vi "AO init.vi"(8 "error in":errorcluster, 9 "Exposure duration specified (s)":dbl=0.5, 10 "Commands in":sgl[](array[numeric]), 11 "Matrix path":path=path "C:/Documents and Settings/User/Desktop/zw/20160113 200nm bead command matrix.aomc") -> (0 "error out":errorcluster, 1 "Camera":T2, 2 "Mirror":T5, 3 "Casao Matrix":T4, 4 "Haso":T3, 5 "Casao":T1)   [LabVIEW 2018]
uses:
  Casao LabVIEW SDK 1.0.5/Drivers_DPhaseModul/PhaseModul.ctl
  Casao LabVIEW SDK 1.0.5/Casao/CasaoMatrix/CasaoMatrix.ctl
  Casao LabVIEW SDK 1.0.5/Haso/Haso/Haso.ctl
  Casao LabVIEW SDK 1.0.5/Haso/Camera/Camera.ctl
  Casao LabVIEW SDK 1.0.5/Casao/Casao/Casao.ctl
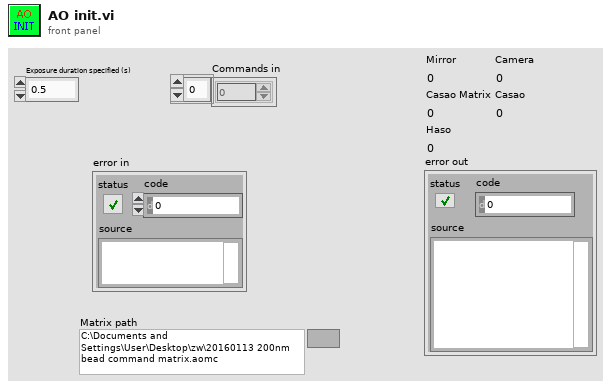
[diagram p1: front panel]
types:
  T1 = typedef "Casao.ctl" = i32
  T2 = typedef "Camera.ctl" = i32
  T3 = typedef "Haso.ctl" = i32
  T4 = typedef "CasaoMatrix.ctl" = i32
  T5 = typedef "PhaseModul.ctl" = i32
  T6 = typedef "Camera preferences.ctl" = cluster{"Exposure duration (µs)":u32, "Exposure duration specified (µs)":u32, "Number of summed images":u32, "Trigger type":enum16{"Internal", "TTL", "Software"}, "Trigger event":enum16{"falling", "rising"}, "Remove background image":bool, "Background image":T7, "Path to background image":string, "Auto exposure":bool, "Auto exposure target (%)":sgl, "Auto exposure tolerance (%)":sgl, "Timeout delay (ms)":u32, "Delay after trigger (µs)":i32}
  T7 = typedef "Image Compat.ctl" = cluster{"Signed/unsigned":bool, "Number of bits":T8, "Internal object id":i32, "Internal data id":i32}
  T8 = typedef "Data alignment enum.ctl" = enum16{"8", "16", "32"}
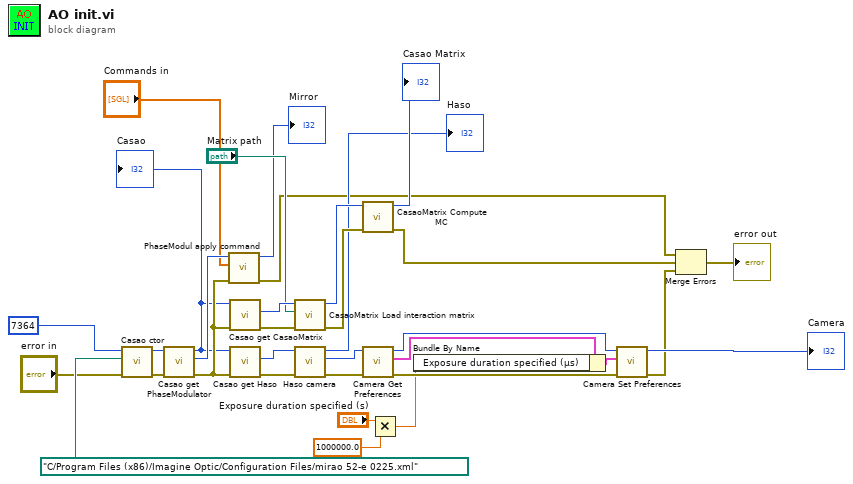
[diagram p0: block diagram]
diagram:
  n1 = call "Casao ctor.vi"("error in (no error)"="error in", "Mirror config file path"=path "C:/Program Files (x86)/Imagine Optic/Configuration Files/mirao 52-e 0225.xml", "Haso serial number"=u32 7364) -> ("error out"=w17:errorcluster, "Casao"=w18:T1)  [unwired: 5 in]
  n2 = call "Casao get PhaseModulator.vi"("error in (no error)"=w17, "Casao"=w18) -> ("error out"=w20:errorcluster, "Mirrror"=w19:T5, "Casao (dup)"=w5:T1)  [unwired: 3 in]
  "Casao" <- w5
  n3 = call "PhaseModul apply command.vi"("error in (no error)"=w20, "Commands in"="Commands in", "Mirror"=w19) -> ("error out"=w9:errorcluster, "Mirror (dup)"=→"Mirror":T5)  [unwired: 2 in, 1 out]
  n4 = call "Casao get CasaoMatrix.vi"("error in (no error)"=w20, "Casao"=w5) -> ("error out"=w33:errorcluster, "Casao matrix"=w32:T4)  [unwired: 3 in, 1 out]
  n5 = call "Casao get Haso.vi"("error in (no error)"=w20, "Casao"=w5) -> ("error out"=w27:errorcluster, "Haso"=w28:T3)  [unwired: 3 in, 1 out]
  n6 = call "CasaoMatrix Load interaction matrix.vi"("error in (no error)"=w33, "Path"="Matrix path", "Casao matrix"=w32) -> ("error out"=w30:errorcluster, "Casao matrix (dup)"=w29:T4)  [unwired: 1 in, 2 out]
  n7 = call "Haso camera.vi"("error in (no error)"=w27, "Haso"=w28) -> ("error out"=w26:errorcluster, "camera"=w25:T2, "Haso (dup)"=→"Haso":T3)  [unwired: 3 in]
  n8 = call "CasaoMatrix Compute MC.vi"("error in (no error)"=w30, "Casao Matrix"=w29) -> ("error out"=w8:errorcluster, "Casao Matrix (dup)"=→"Casao Matrix":T4)  [unwired: 4 in]
  n9 = call "Camera Get Preferences.vi"("error in (no error)"=w26, "Camera"=w25) -> ("error out"=w24:errorcluster, "Camera Preferences"=w23:T6, "Camera (dup)"=w22:T2)  [unwired: 3 in]
  n10 = Multiply(x="Exposure duration specified (s)", y=1000000.0) -> (x*y=w3:dbl)
  n11 = Bundle By Name(cluster=w23, "Exposure duration specified (µs)"=w3) -> (w21:T6)
  n12 = call "Camera Set Preferences.vi"("error in (no error)"=w24, "Camera Preferences"=w21, "Camera"=w22) -> ("error out"=w4:errorcluster, "Camera (dup)"=→"Camera":T2)  [unwired: 3 in]
  n13 = Merge Errors(w9, w8, w4) -> (→"error out":errorcluster)
